vi "HP 5890 Data Acquisition.vi"() -> ()   [LabVIEW 2010]
uses:
  signal.ctl
  detector.ctl
  zones.ctl
  toolbar icons/log data.ctl
  toolbar icons/data not logging.ctl
  toolbar icons/file comment.ctl
  state.ctl
panel:
  out "Detectors 2":T1={"Det A"="FID", "Det B"="TCD"}
  out "zones 2":T2={"Inj A zone"=TRUE, "Det A zone"=TRUE, "Inj B zone"=TRUE, "Det B zone"=TRUE}
  out "state":T3
  out "refnum":refnum<file>
  out "Valid File":bool
  in  "File Comment":T4
  out "file warning":T5
  in  "Log Data":T6
  out "Quiting":bool
  out "Chart":dbl[](graph)
  in  "Quit":bool
  in  "Set method":bool
  in  "Measure Sample":bool
  out "zones":T2={"Inj A zone"=TRUE, "Det A zone"=TRUE, "Inj B zone"=TRUE, "Det B zone"=TRUE}
  out "Detectors":T1={"Det A"="FID", "Det B"="TCD"}
  out "Det in use":string
  out "measure sample":bool
  out "method set":bool
  out "data points":u8
  out "delta x":dbl=0.05 format="%.2f"
  out "Signal 1":T7
  out "signals":enum16{"signal 1", "signals 1 and 2"}(ring)=enum."signals 1 and 2"
  in  "Serial Port":refnum<visa-resource-name>="COM1"
  # "s"
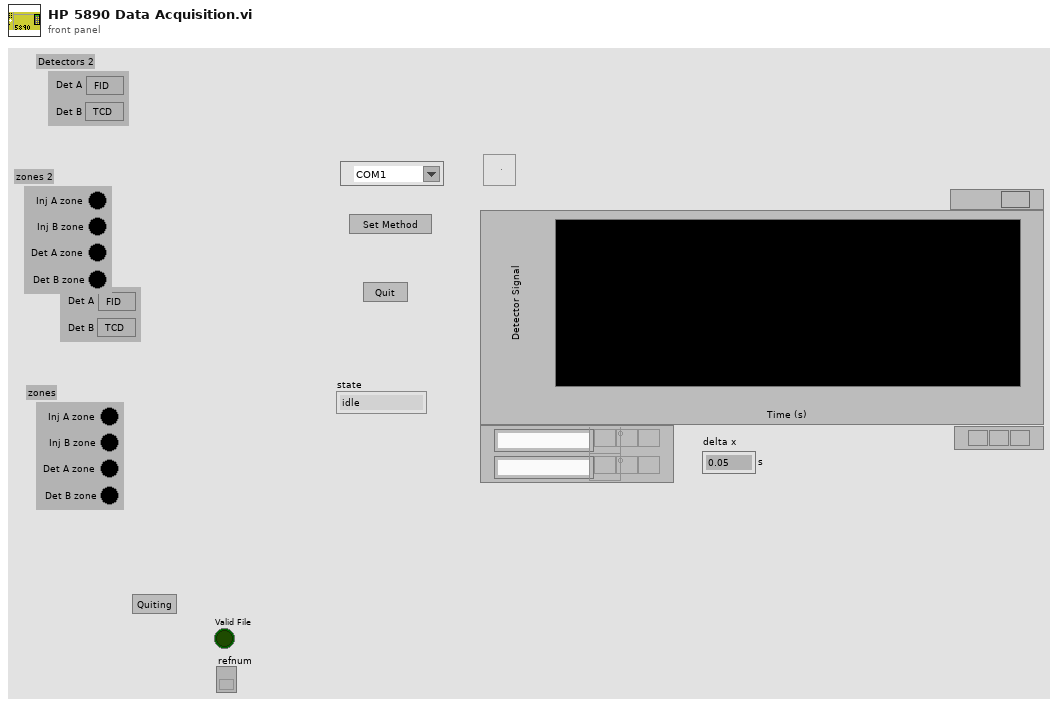
[diagram p1: front panel]
types:
  T1 = typedef "detector.ctl" = cluster{"Det A":string, "Det B":string}
  T2 = typedef "zones.ctl" = cluster{"Inj A zone":bool, "Det A zone":bool, "Inj B zone":bool, "Det B zone":bool}
  T3 = typedef "state.ctl" = enum16{"idle", "initialize sample", "sample", "finish sample", "Quit"}
  T4 = typedef "file comment.ctl" = bool
  T5 = typedef "data not logging.ctl" = bool
  T6 = typedef "log data.ctl" = bool
  T7 = typedef "signal.ctl" = enum16{"Detector A", "Detector B", "Oven temperature", "Comp 1", "Comp 2", "Inlet A temperature", "Inlet B temperature", "Detector A temperature", "Detector B temperature", "Test Signal"}
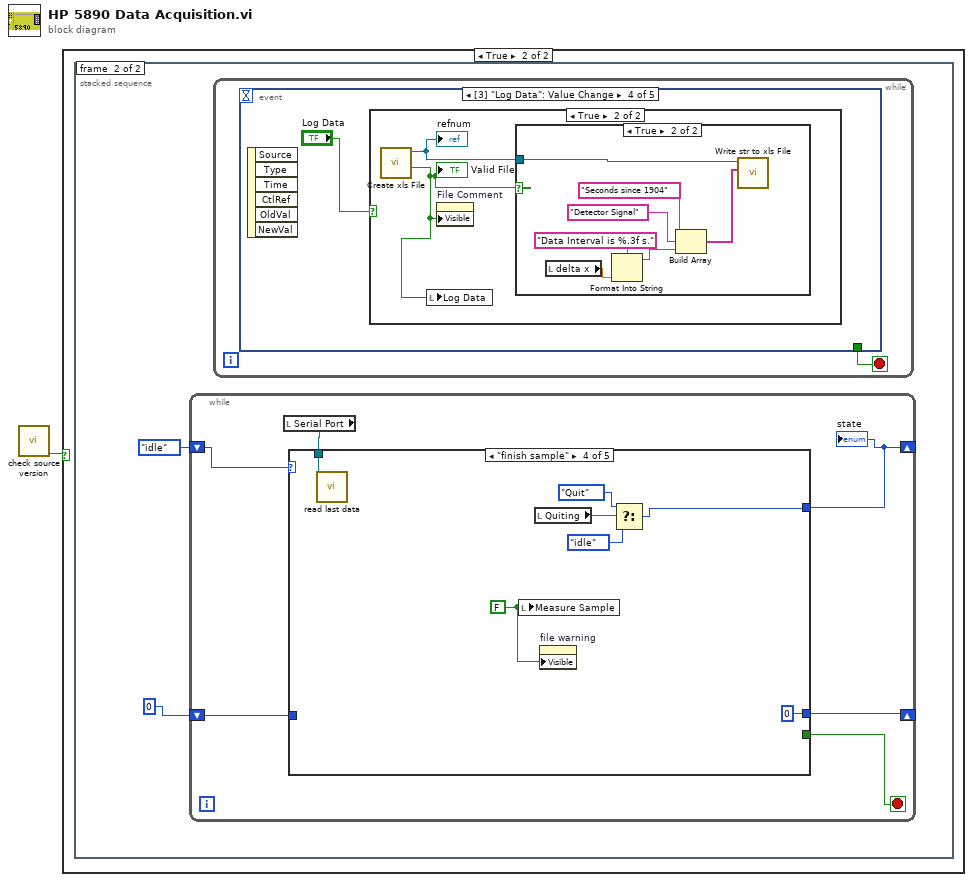
[diagram p0: block diagram]
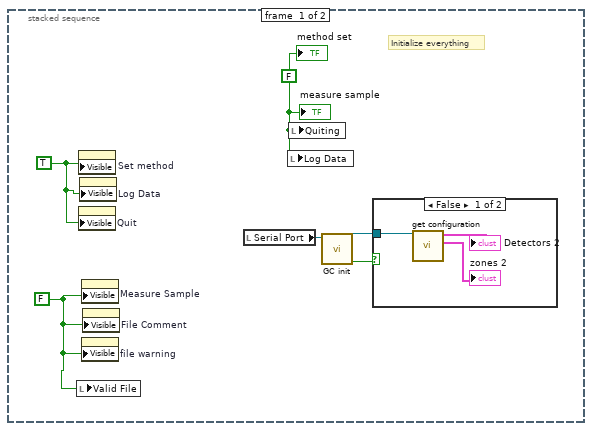
[diagram p3: hidden frame]
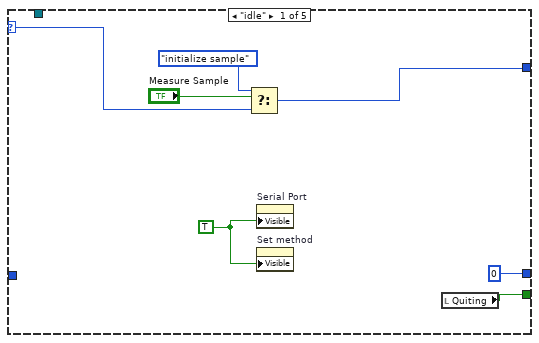
[diagram p5: hidden frame]
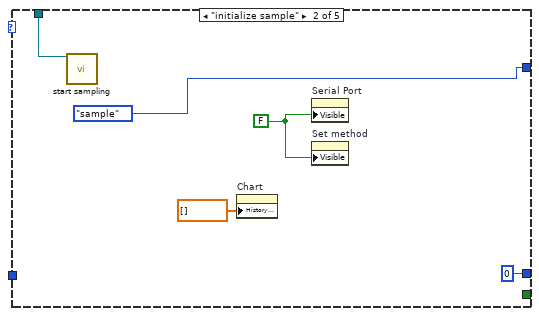
[diagram p6: hidden frame]
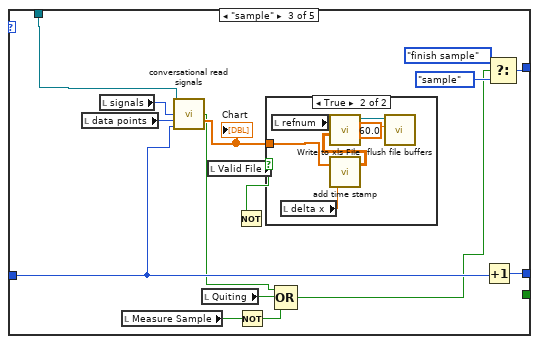
[diagram p7: hidden frame]
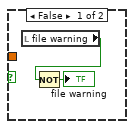
[diagram p8: hidden frame]
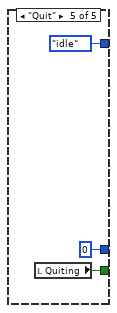
[diagram p9: hidden frame]
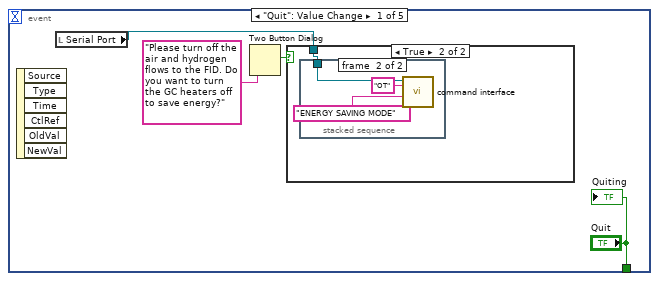
[diagram p10: hidden frame]
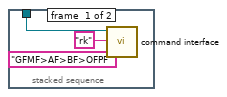
[diagram p12: hidden frame]
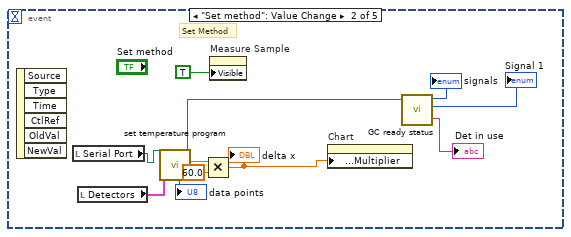
[diagram p13: hidden frame]
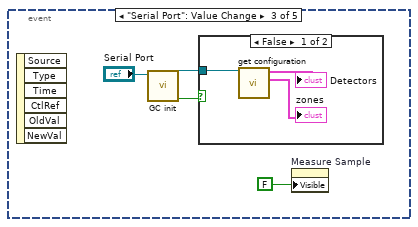
[diagram p14: hidden frame]
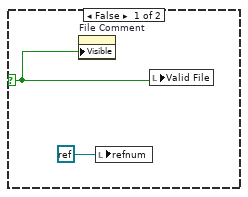
[diagram p16: hidden frame]
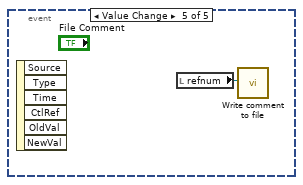
[diagram p18: hidden frame]
diagram:
  n1 = call "check source version.vi"() -> ("continue running?"=w1:bool)  [unwired: 2 in, 3 out]
  n2 = case shown="True" w1 {
    frame False {
    }
    frame True {
      n3 = stacked-sequence {
        frame #0 {
          w2 = FALSE
          w7 = TRUE
          w3 = FALSE
          # "Initialize everything"
          n4 = local write "Valid File"(w2) -> ()
          n5 = property on="Set method" class="Bool"("Visible"=w7) -> ()  [unwired: 2 in, 2 out]
          n6 = property on="Quit" class="Bool"("Visible"=w7) -> ()  [unwired: 2 in, 2 out]
          n7 = property on="Log Data" class="Bool (strict)"("Visible"=w7) -> ()  [unwired: 2 in, 2 out]
          n8 = property on="Measure Sample" class="Bool (strict)"("Visible"=w2) -> ()  [unwired: 2 in, 2 out]
          n9 = property on="file warning" class="Bool"("Visible"=w2) -> ()  [unwired: 2 in, 2 out]
          n10 = property on="File Comment" class="Bool"("Visible"=w2) -> ()  [unwired: 2 in, 2 out]
          n11 = local read "Serial Port"() -> (w4:refnum<visa-resource-name>)
          n12 = local write "Log Data"(w3) -> ()
          n13 = local write "Quiting"(w3) -> ()
          n14 = call "GC init.vi"("Serial Port"=w4) -> ("error"=w5:bool, "Serial Port"=w6:refnum<visa-resource-name>)  [unwired: 9 in]
          n15 = case shown="False" w5 {
            tunnel: w6 -> [w10 _]
            frame False {
              n16 = call "get configuration.vi"("Serial Port"=w10) -> ("zones"=→"zones 2":T2, "Detectors"=→"Detectors 2":T1)  [unwired: 5 in, 1 out]
            }
            frame True {
            }
          }
          "method set" <- w3
          "measure sample" <- w3
        }
        frame #1 {
          n17 = while {
            shift-right: [w16] -> _
            shift-left: state."idle" ("state") -> [w17]
            shift-right: [w14] -> _
            shift-left: 0 -> [w13]
            stop <- w15 stop-if-true
            n18 = local read "Serial Port"() -> (w18:refnum<visa-resource-name>)
            n19 = case shown="\"finish sample\"" w17 {
              tunnel: w18 -> [_ w30 w45 w60 _]
              selector: w17 -> [w24 _ _ _ _]
              tunnel: [w23 state."sample" ("f") w44 w56 state."idle" ("f")] -> w16
              tunnel: [w19 _ _ _ w63] -> w15
              tunnel: [0 0 w38 0 0] -> w14
              tunnel: w13 -> [_ _ w37 _ _]
              frame "idle" {
                w20 = TRUE
                n20 = Select(t=state."initialize sample", s="Measure Sample", f=w24) -> (s? t:f=w23:T3)
                n21 = property on="Serial Port" class="VISAName"("Visible"=w20) -> ()  [unwired: 2 in, 2 out]
                n22 = property on="Set method" class="Bool"("Visible"=w20) -> ()  [unwired: 2 in, 2 out]
                n23 = local read "Quiting"() -> (w19:bool)
              }
              frame "initialize sample" {
                w26 = FALSE
                n24 = call "start sampling.vi"("Serial Port"=w30) -> ()  [unwired: 14 in, 1 out]
                n25 = property on="Chart" class="WFChart (strict)"("History Data"=dbl[] []) -> ()  [unwired: 2 in, 2 out]
                n26 = property on="Serial Port" class="VISAName"("Visible"=w26) -> ()  [unwired: 2 in, 2 out]
                n27 = property on="Set method" class="Bool"("Visible"=w26) -> ()  [unwired: 2 in, 2 out]
              }
              frame "sample" {
                n28 = local read "data points"() -> (w43:u8)
                n29 = local read "signals"() -> (w42:enum16{"signal 1", "signals 1 and 2"})
                n30 = local read "Measure Sample"() -> (w34:bool)
                n31 = call "conversational read signals.vi"("Serial Port"=w45, "signals"=w42, "data points"=w43, "i"=w37) -> ("run done"=w36:bool, "signal 1"=w41:dbl[])  [unwired: 5 in, 5 out]
                "Chart" <- w41
                n32 = local read "Quiting"() -> (w35:bool)
                n33 = local read "Valid File"() -> (w31:bool)
                n34 = Not(x=w31) -> ()  [unwired: 1 out]
                n35 = Not(x=w34) -> (.not. x?=w32:bool)
                n36 = case shown="True" w31 {
                  tunnel: w41 -> [_ w50]
                  frame False {
                    n37 = local read "file warning"() -> (w47:T5)
                    n38 = Not(x=w47) -> (.not. x?=→"file warning":T5)
                  }
                  frame True {
                    n39 = local read "refnum"() -> (w53:refnum<file>)
                    n40 = local read "delta x"() -> (w48:dbl)
                    n41 = call "add time stamp.vi"("delta x"=w48, "signal 1"=w50) -> ("Data w time"=w49:ext[][])  [unwired: 1 in]
                    n42 = call "Write to xls File.vi"("2D data"=w49, "refnum"=w53) -> ("dup refnum"=w52:refnum<file>)  [unwired: 8 in, 1 out]
                    n43 = call "flush file buffers.vi"("Flush interval (s)"=60.0, "refnum"=w52) -> ()  [unwired: 8 in, 2 out]
                  }
                }
                n44 = Compound Arithmetic op=OR(w36, w35, w32) -> (w33:bool)
                n45 = Increment(x=w37) -> (x+1=w38:i32)
                n46 = Select(t=state."finish sample" ("f"), s=w33, f=state."sample") -> (s? t:f=w44:T3)
              }
              frame "finish sample" {
                w54 = FALSE ("Measure Sample")
                n47 = call "read last data.vi"("Serial Port"=w60) -> ()  [unwired: 9 in, 2 out]
                n48 = local write "Measure Sample"(w54) -> ()
                n49 = local read "Quiting"() -> (w59:bool)
                n50 = property on="file warning" class="Bool"("Visible"=w54) -> ()  [unwired: 2 in, 2 out]
                n51 = Select(t=state."Quit" ("f"), s=w59, f=state."idle") -> (s? t:f=w56:T3)
              }
              frame "Quit" {
                n52 = local read "Quiting"() -> (w63:bool)
              }
            }
            "state" <- w16
          }
          n53 = while {
            stop <- w64 stop-if-true
            n54 = event shown="[3] \"Log Data\": Value Change" {
              selector: _ -> [_ _ _ _ _]
              dyn-events: _ -> [_ _ _ _ _]
              timeout: _ -> [_ _ _ _ _]
              tunnel: ["Quit" _ _ _ _] -> w64
              event "Quit": Value Change {
                n55 = event-data() -> ()  [unwired: 1 in, 6 out]
                n56 = local read "Serial Port"() -> (w65:refnum<visa-resource-name>)
                n57 = Two Button Dialog(message="Please turn off the air and hydrogen flows to the FID. Do you want to turn the GC heaters off to save energy?") -> (T button?=w66:bool)  [unwired: 2 in]
                n58 = case shown="True" w66 {
                  tunnel: w65 -> [_ w69]
                  frame False {
                  }
                  frame True {
                    n59 = stacked-sequence {
                      tunnel: w69 -> [w72 w73]
                      frame #0 {
                        n60 = call "command interface.vi"("Parameter"="GFMF>AF>BF>OFPF", "command"="rk", "Serial Port"=w72) -> ()  [unwired: 4 in, 4 out]
                      }
                      frame #1 {
                        n61 = call "command interface.vi"("Parameter"="ENERGY SAVING MODE", "command"="OT", "Serial Port"=w73) -> ()  [unwired: 4 in, 4 out]
                      }
                    }
                  }
                }
                "Quiting" <- "Quit"
              }
              event "Set method": Value Change {
                # "Set Method"
                n62 = event-data() -> ()  [unwired: 1 in, 6 out]
                n63 = local read "Serial Port"() -> (w78:refnum<visa-resource-name>)
                n64 = local read "Detectors"() -> (w84:T1)
                n65 = call "set temperature program.vi"("Detectors"=w84, "Serial Port"=w78) -> ("delta x"=w80:dbl, "Serial Port"=w81:refnum<visa-resource-name>, "data points"=→"data points":u8)  [unwired: 5 in, 2 out]
                n66 = Multiply(x=w80, y=60.0) -> (x*y=w76:dbl)
                "delta x" <- w76
                n67 = property on="Measure Sample" class="Bool (strict)"("Visible"=TRUE) -> ()  [unwired: 2 in, 2 out]
                n68 = property on="Chart" class="WFChart (strict)"("X Scale.Offset and Multiplier:Multiplier"=w76) -> ()  [unwired: 2 in, 2 out]
                n69 = call "GC ready status.vi"("Serial Port"=w81) -> ("signals"=→"signals":enum16{"signal 1", "signals 1 and 2"}, "Signal 1"=→"Signal 1":T7, "Det in use"=→"Det in use":string)  [unwired: 4 in, 3 out]
              }
              event "Serial Port": Value Change {
                n70 = event-data() -> ()  [unwired: 1 in, 6 out]
                n71 = call "GC init.vi"("Serial Port"="Serial Port") -> ("error"=w89:bool, "Serial Port"=w90:refnum<visa-resource-name>)  [unwired: 9 in]
                n72 = case shown="False" w89 {
                  tunnel: w90 -> [w93 _]
                  frame False {
                    n73 = call "get configuration.vi"("Serial Port"=w93) -> ("zones"=→"zones":T2, "Detectors"=→"Detectors":T1)  [unwired: 5 in, 1 out]
                  }
                  frame True {
                  }
                }
                n74 = property on="Measure Sample" class="Bool (strict)"("Visible"=FALSE) -> ()  [unwired: 2 in, 2 out]
              }
              event Value Change {
                n75 = event-data() -> ()  [unwired: 1 in, 6 out]
                n76 = case shown="True" "Log Data" {
                  selector: "Log Data" -> [w96 _]
                  frame False {
                    n77 = property on="File Comment" class="Bool"("Visible"=w96) -> ()  [unwired: 2 in, 2 out]
                    n78 = local write "refnum"(refnum<k0> refnum) -> ()
                    n79 = local write "Valid File"(w96) -> ()
                  }
                  frame True {
                    n80 = call "Create xls File.vi"() -> ("Valid File"=w97:bool, "refnum"=w98:refnum<file>)  [unwired: 4 in, 2 out]
                    "Valid File" <- w97
                    "refnum" <- w98
                    n81 = local write "Log Data"(w97) -> ()
                    n82 = property on="File Comment" class="Bool"("Visible"=w97) -> ()  [unwired: 2 in, 2 out]
                    n83 = case shown="True" w97 {
                      tunnel: w98 -> [_ w105]
                      frame False {
                      }
                      frame True {
                        n84 = local read "delta x"() -> (w103:dbl)
                        n85 = Format Into String(format string="Data Interval is %.3f s.", w103) -> (resulting string=w102:string)  [unwired: 2 in, 1 out]
                        n86 = Build Array("Seconds since 1904", "Detector Signal" ("string"), w102) -> (w99:string[])
                        n87 = call "Write str to xls File.vi"("1D data"=w99, "refnum"=w105) -> ()  [unwired: 8 in, 2 out]
                      }
                    }
                  }
                }
              }
              event Value Change {
                n88 = event-data() -> ()  [unwired: 1 in, 6 out]
                n89 = local read "refnum"() -> (w106:refnum<file>)
                n90 = call "Write comment to file.vi"("refnum"=w106) -> ()  [unwired: 7 in, 2 out]
              }
            }
          }
        }
      }
    }
  }
